vi "ButtonHold3Totes.vi"(11 "Buttons":bool[](array[boolean])) -> (3 "Boolean":bool)   [LabVIEW 2014]
uses:
  Gantry/GantryGlobals.vi
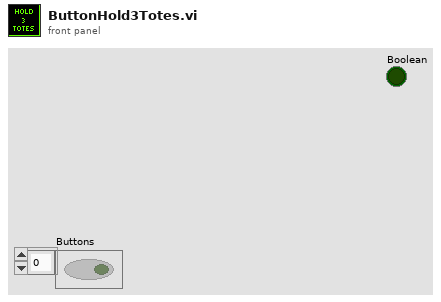
[diagram p1: front panel]
types:
  T1 = enum16{"WaitForInput", "LowerLift", "OpenArms", "RaiseLift", "CloseArms"}
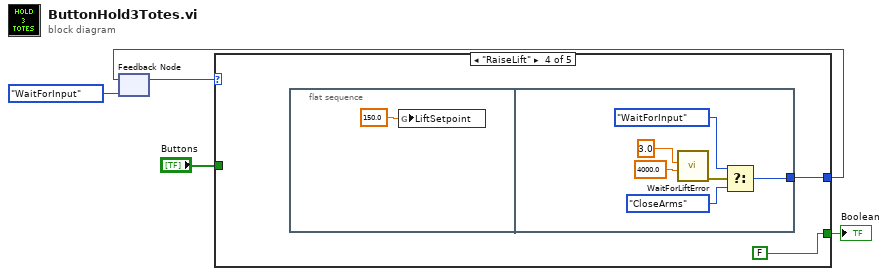
[diagram p0: block diagram]
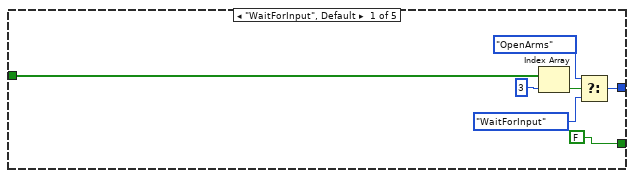
[diagram p2: hidden frame]
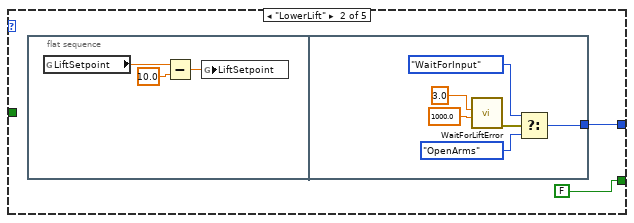
[diagram p3: hidden frame]
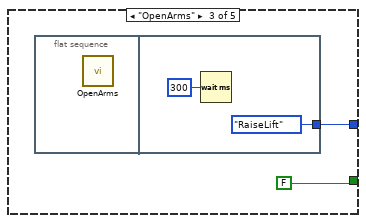
[diagram p4: hidden frame]
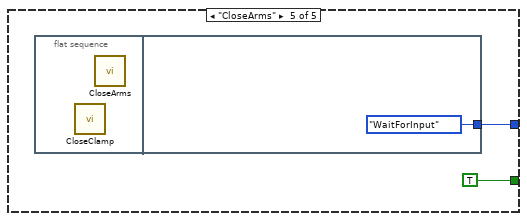
[diagram p5: hidden frame]
diagram:
  n1 = feedback #1(T1."WaitForInput" ("Enum")) -> (w2:T1)
  n2 = case shown="\"RaiseLift\"" w2 {
    tunnel: [w11 w14 w25 w29 w38] -> w4
    tunnel: "Buttons" -> [w9 _ _ _ _]
    tunnel: [FALSE FALSE FALSE FALSE TRUE] -> w1
    frame "WaitForInput", Default {
      n3 = Index Array(array=w9, index=3) -> (element=w7:bool)
      n4 = Select(t=T1."OpenArms" ("Enum"), s=w7, f=T1."WaitForInput" ("Enum")) -> (s? t:f=w11:T1)
    }
    frame "LowerLift" {
      n5 = flat-sequence {
        tunnel: [w18] -> w14
        frame #0 {
          n6 = global read "GantryGlobals.vi" "LiftSetpoint"() -> (w17:dbl)
          n7 = Subtract(x=w17, y=10.0) -> (x-y=w16:dbl)
          n8 = global write "GantryGlobals.vi" "LiftSetpoint"(w16) -> ()
        }
        frame #1 {
          n9 = call "WaitForLiftError.vi"("Timeout (ms)"=1000.0, "AllowedError"=3.0) -> ("error out"=w23:errorcluster)  [unwired: 9 in]
          n10 = Select(t=T1."WaitForInput" ("Enum"), s=w23, f=T1."OpenArms" ("Enum")) -> (s? t:f=w18:T1)
        }
      }
    }
    frame "OpenArms" {
      n11 = flat-sequence {
        tunnel: [T1."RaiseLift" ("Enum")] -> w25
        frame #0 {
          n12 = call "OpenArms.vi"() -> ()  [unwired: 12 in]
        }
        frame #1 {
          n13 = Wait (ms)(milliseconds to wait=u32 300) -> ()  [unwired: 1 out]
        }
      }
    }
    frame "RaiseLift" {
      n14 = flat-sequence {
        tunnel: [w31] -> w29
        frame #0 {
          n15 = global write "GantryGlobals.vi" "LiftSetpoint"(150.0 ("LiftSetpoint")) -> ()
        }
        frame #1 {
          n16 = call "WaitForLiftError.vi"("Timeout (ms)"=4000.0, "AllowedError"=3.0) -> ("error out"=w36:errorcluster)  [unwired: 9 in]
          n17 = Select(t=T1."WaitForInput" ("Enum"), s=w36, f=T1."CloseArms" ("Enum")) -> (s? t:f=w31:T1)
        }
      }
    }
    frame "CloseArms" {
      n18 = flat-sequence {
        tunnel: [T1."WaitForInput" ("Enum")] -> w38
        frame #0 {
          n19 = call "CloseClamp.vi"() -> ()  [unwired: 12 in]
          n20 = call "CloseArms.vi"() -> ()  [unwired: 12 in]
        }
        frame #1 {
        }
      }
    }
  }
  "Boolean" <- w1
  n21 = feedback-in #1(w4) -> ()
